vi "FMDemod_COM(SubVI).vi"(9 "QSamples":dbl[](array[numeric]), 10 "ISamples":dbl[](array[numeric]), 11 "FMDemodRTLSDR_COM.IClass1":refnum<k7>) -> (3 "Baseband":dbl[](array[numeric]))   [LabVIEW 2013]
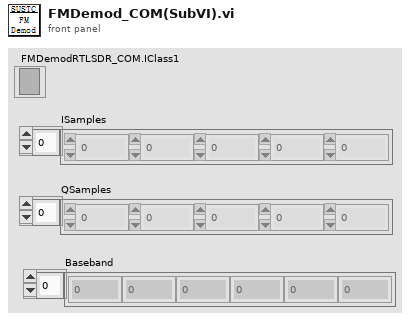
[diagram p1: front panel]
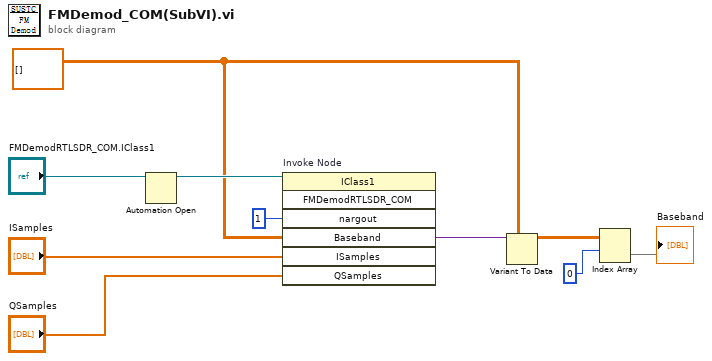
[diagram p0: block diagram]
diagram:
  w1 = dbl[][] []
  n1 = Automation Open(Automation Refnum="FMDemodRTLSDR_COM.IClass1") -> (Automation Refnum=w6:refnum<k7>)  [unwired: 3 in, 1 out]
  n2 = invoke on="Invoke Node" class="IClass1" method="FMDemodRTLSDR_COM"(reference=w6, "nargout"=1, "Baseband"=w1, "ISamples"="ISamples", "QSamples"="QSamples") -> ("Baseband"=w10:variant)  [unwired: 2 in, 6 out]
  n3 = Variant To Data(type=w1, Variant=w10) -> (data=w4:dbl[][])  [unwired: 1 in, 1 out]
  n4 = Index Array(array=w4, index (row)=0) -> (element=→"Baseband":dbl[])  [unwired: 1 in]
